vi "_5Basic_Gates.vi"() -> ()   [LabVIEW 2018]
panel:
  out "LED3":bool
  out "LED2":bool
  out "LED1":bool
  in  "NOT":bool
  in  "Or2":bool
  in  "Or1":bool
  in  "Ai2":bool
  in  "Ai1":bool
  # "AND Logic"
  # "OR Logic"
  # "NOT Logic"
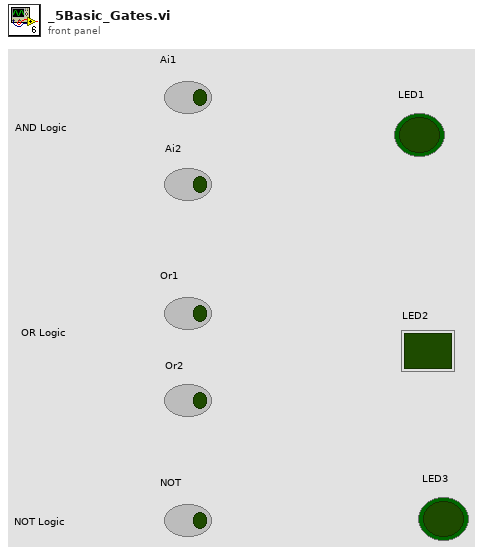
[diagram p1: front panel]
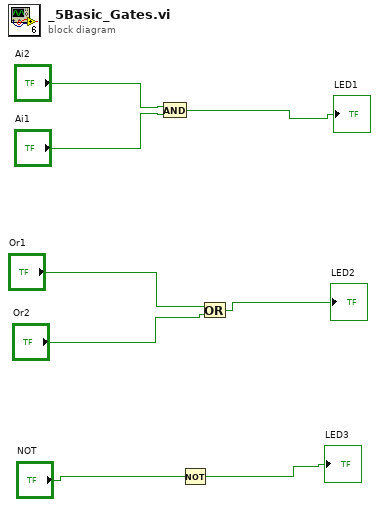
[diagram p0: block diagram]
diagram:
  n1 = And(x="Ai2", y="Ai1") -> (x .and. y?=→"LED1":bool)
  n2 = Not(x="NOT") -> (.not. x?=→"LED3":bool)
  n3 = Or(x="Or1", y="Or2") -> (x .or. y?=→"LED2":bool)
